vi "整点（时分秒）闹钟.vi"(8 "Error In":errorcluster caption="错误输入", 9 "模式":enum16{"秒", "分", "时"}(ring)) -> (0 "Error Out":errorcluster caption="错误输出", 1 "时刻":i32, 3 "时间到":bool)   [LabVIEW 2012]
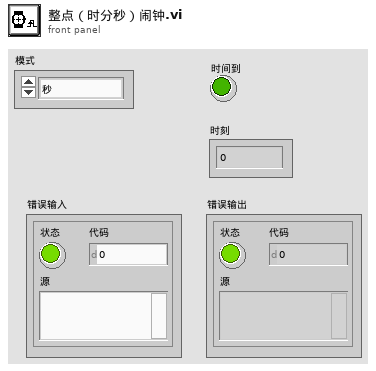
[diagram p1: front panel]
types:
  T1 = typedef "LVDateTimeRec.ctl" = cluster{"秒数的小数部分":dbl, "秒":i32, "分":i32, "时":i32, "日":i32, "月":i32, "年":i32, "天数（周）":i32, "天数（年）":i32, "DST":i32}
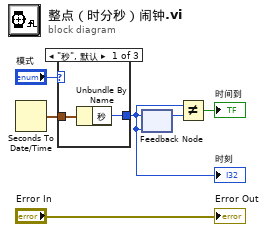
[diagram p0: block diagram]
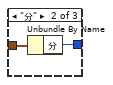
[diagram p2: hidden frame]
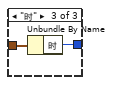
[diagram p3: hidden frame]
diagram:
  n1 = Seconds To Date/Time() -> (date time rec=w4:T1)  [unwired: 2 in]
  n2 = case shown="\"秒\", 默认" "模式" {
    tunnel: w4 -> [w8 w10 w12]
    tunnel: [w7 w9 w11] -> w2
    frame "秒", Default {
      n3 = Unbundle By Name(w8) -> ("秒"=w7:i32)
    }
    frame "分" {
      n4 = Unbundle By Name(w10) -> ("分"=w9:i32)
    }
    frame "时" {
      n5 = Unbundle By Name(w12) -> ("时"=w11:i32)
    }
  }
  "时刻" <- w2
  n6 = feedback #1(w2) -> (w3:i32)
  n7 = feedback-in #1(w2) -> ()
  n8 = Not Equal?(x=w2, y=w3) -> (x != y?=→"时间到":bool)
  "Error Out" <- "Error In"
